vi "Simple Counter with Reset.vi"(2 "Add":bool, 3 "Reset":bool) -> (0 "Loop Counter":u64, 1 "Last Count Before Reset":u64)   [LabVIEW 2009]
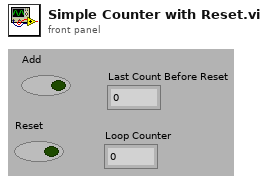
[diagram p1: front panel]
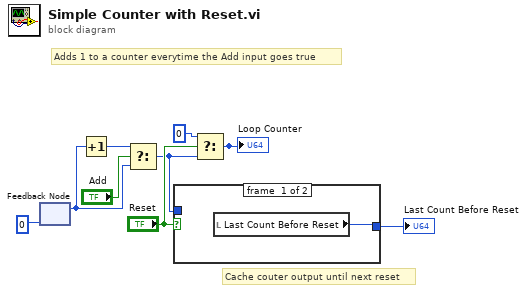
[diagram p0: block diagram]
diagram:
  # "Adds 1 to a counter everytime the Add input goes true"
  # "Cache couter output until next reset"
  n1 = feedback #1(u64 0) -> (w5:u64)
  n2 = Increment(x=w5) -> (x+1=w6:u64)
  n3 = Select(t=w6, s="Add", f=w5) -> (s? t:f=w2:u64)
  n4 = case shown="False" "Reset" {
    tunnel: w2 -> [_ w11]
    tunnel: [w10 w11] -> w1
    frame #0 {
      n5 = local read "Last Count Before Reset"() -> (w10:u64)
    }
    frame #1 {
    }
  }
  "Last Count Before Reset" <- w1
  n6 = Select(t=u64 0, s="Reset", f=w2) -> (s? t:f=w3:u64)
  "Loop Counter" <- w3
